vi "GetPowerLineConfig.vi"(9 "Power Line\nIdentifier":T2) -> (3 "Power Line\nConfiguration":T1 {"Max Current [A]" format="%#_13g"; "Min Current [A]" format="%#_13g"; "Shunt Resistor [Ohm]" format="%#_13g"})   [LabVIEW 2020]
uses:
  PowerLineId.ctl
  PowerLineConfig.ctl
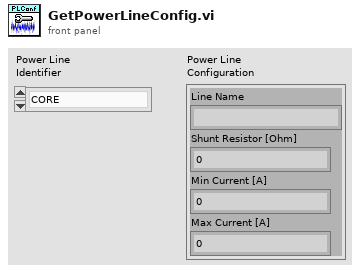
[diagram p1: front panel]
types:
  T1 = typedef "PowerLineConfig.ctl" = cluster{"Line Name":string, "Shunt Resistor [Ohm]":dbl, "Min Current [A]":dbl, "Max Current [A]":dbl}
  T2 = typedef "PowerLineId.ctl" = enum8{"CORE", "DDR_SOC", "IO", "PLL", "PCIEVP", "PCIEVPH", "DDR_MEM", "DDR_PLL", "DDR_VPP"}
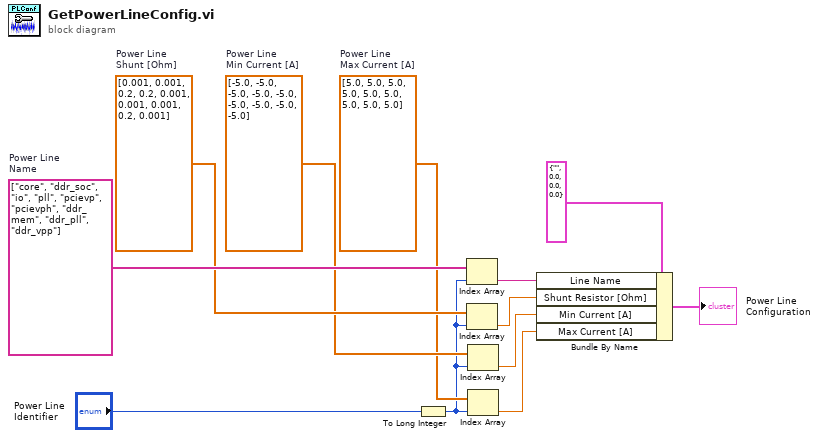
[diagram p0: block diagram]
diagram:
  w7 = dbl[] [5.0, 5.0, 5.0, 5.0, 5.0, 5.0, 5.0, 5.0, 5.0]  # Power Line Max Current [A]
  w8 = dbl[] [-5.0, -5.0, -5.0, -5.0, -5.0, -5.0, -5.0, -5.0, -5.0]  # Power Line Min Current [A]
  w9 = dbl[] [0.001, 0.001, 0.2, 0.2, 0.001, 0.001, 0.001, 0.2, 0.001]  # Power Line Shunt [Ohm]
  w10 = string[] ["core", "ddr_soc", "io", "pll", "pcievp", "pcievph", "ddr_mem", "ddr_pll", "ddr_vpp"]  # Power Line Name
  n1 = To Long Integer(number="Power Line\nIdentifier") -> (32bit integer=w6:i32)
  n2 = Index Array(array=w10, index=w6) -> (element=w5:string)
  n3 = Index Array(array=w9, index=w6) -> (element=w4:dbl)
  n4 = Index Array(array=w8, index=w6) -> (element=w3:dbl)
  n5 = Index Array(array=w7, index=w6) -> (element=w2:dbl)
  n6 = Bundle By Name(cluster=T1 {"Line Name"="", "Shunt Resistor [Ohm]"=0.0, "Min Current [A]"=0.0, "Max Current [A]"=0.0} ("HiFive Unmatched\nPower Monitor Line Configuration"), "Line Name"=w5, "Shunt Resistor [Ohm]"=w4, "Min Current [A]"=w3, "Max Current [A]"=w2) -> (→"Power Line\nConfiguration":T1)
